vi "Create Data Log.vi"(8 "error in (no error)":errorcluster, 11 "Model in":refnum<class "Model.lvclass">) -> (0 "error out":errorcluster, 3 "Model out":refnum<class "Model.lvclass">)   [LabVIEW 2016, in "Model.lvclass"]
uses:
  Model.lvclass
  Typedefs/TestLogTypes.ctl
  Test Log/Test Log Factory/OperationsLogFactory.lvclass
  Model.lvclass/Model.ctl
  Test Log/Test Log/OperationsLog.lvclass
  Typedefs/M1M3SupportEUI_TypeDefs.lvlib
panel:
  in  "error in (no error) 2":errorcluster
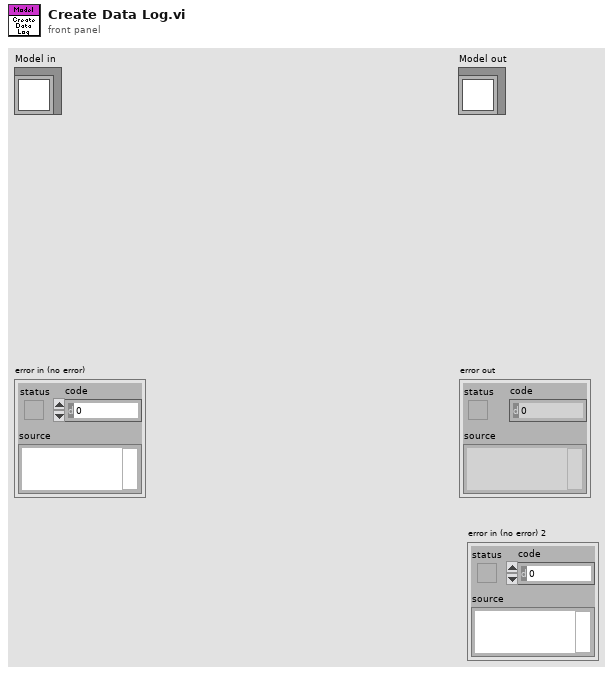
[diagram p1: front panel]
types:
  T1 = typedef "M1M3SupportEUI_TypeDefs.lvlib/TestLogTypes.ctl" = enum16{"CSV Test Log"}
  T2 = typedef "M1M3SupportEUI_TypeDefs.lvlib/TestSettings.ctl" = cluster{"Operator":string}
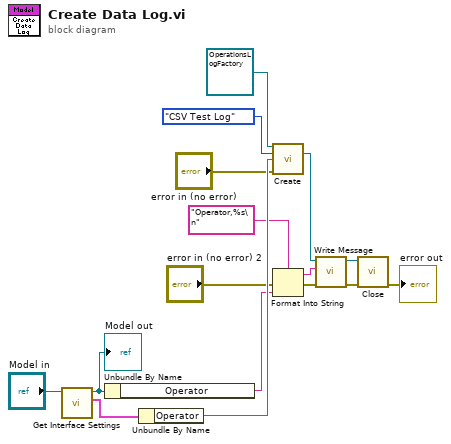
[diagram p0: block diagram]
diagram:
  n1 = call "Get Interface Settings.vi"("Model in"="Model in") -> ("Interface Settings"=w14:T2, "Model out"=w4:refnum<class "Model.lvclass">)  [unwired: 9 in]
  "Model out" <- w4
  n2 = Unbundle By Name(w4) -> ("Operator"=w9:string)
  n3 = Unbundle By Name(w14) -> ("Operator"=w16:string)
  n4 = call-dynamic "Create.vi"("Test Log Factory in"=refnum<class "OperationsLogFactory.lvclass"> refnum ("Test Log Factory.lvclass"), "Test Log Types"=TestLogTypes."CSV Test Log" ("TestLogTypes"), "Test Name"=w16, "error in (no error)"="error in (no error)") -> ("Test Log"=w5:refnum<class "OperationsLog.lvclass">)  [unwired: 9 in, 2 out]
  n5 = Format Into String(format string="Operator,%s\n", error in="error in (no error) 2", w9) -> (resulting string=w6:string, error out=w7:errorcluster)  [unwired: 1 in]
  n6 = call-dynamic "Write Message.vi"("error in (no error)"=w7, "Message"=w6, "Test Log in"=w5) -> ("error out"=w1:errorcluster, "Test Log out"=w2:refnum<class "OperationsLog.lvclass">)  [unwired: 7 in]
  n7 = call-dynamic "Close.vi"("error in (no error)"=w1, "Test Log in"=w2) -> ("error out"=→"error out":errorcluster)  [unwired: 8 in, 1 out]
